vi "acquire multi init subvi ch2.vi"(8 "错误输入（无错误）":errorcluster caption="error in（no error）", 11 "VISA resource name":refnum<visa-resource-name>) -> (0 "错误输出":errorcluster caption="error out", 2 "read buffer":string, 3 "VISA resource name out":refnum<visa-resource-name>)   [LabVIEW 2023, in "owon.lvlib"]
uses:
  owon.lvlib
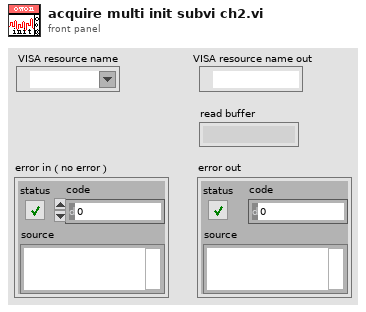
[diagram p1: front panel]
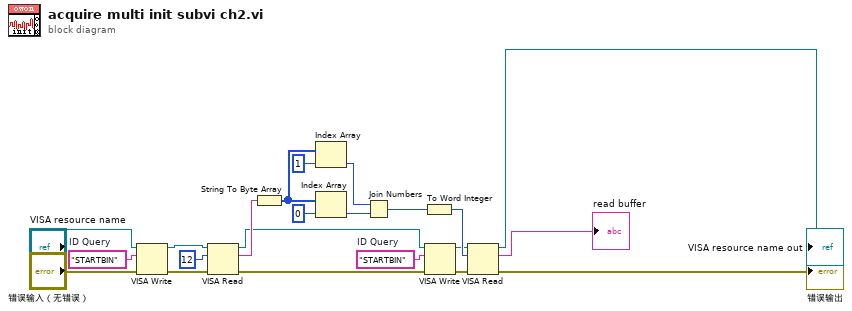
[diagram p0: block diagram]
diagram:
  w14 = "STARTBIN"  # ID Query
  w6 = "STARTBIN"  # ID Query
  n1 = VISA Write(VISA resource name="VISA resource name", write buffer=w14, error in (no error)="错误输入（无错误）") -> (VISA resource name out=w10:refnum<visa-resource-name>, error out=w11:errorcluster)  [unwired: 1 out]
  n2 = VISA Read(VISA resource name=w10, byte count=u32 12, error in (no error)=w11) -> (VISA resource name out=w7:refnum<visa-resource-name>, read buffer=w21:string, error out=w8:errorcluster)  [unwired: 1 out]
  n3 = String To Byte Array(string=w21) -> (unsigned byte array=w16:u8[])
  n4 = Index Array(array=w16, index=1 ("索引")) -> (element=w18:u8)
  n5 = Index Array(array=w16, index=0 ("索引")) -> (element=w19:u8)
  n6 = Join Numbers(hi=w18, lo=w19) -> ((hi.lo)=w20:u16)
  n7 = To Word Integer(number=w20) -> (16bit integer=w22:i16)
  n8 = VISA Write(VISA resource name=w7, write buffer=w6, error in (no error)=w8) -> (VISA resource name out=w3:refnum<visa-resource-name>, error out=w4:errorcluster)  [unwired: 1 out]
  n9 = VISA Read(VISA resource name=w3, byte count=w22, error in (no error)=w4) -> (VISA resource name out=→"VISA resource name out":refnum<visa-resource-name>, read buffer=→"read buffer":string, error out=→"错误输出":errorcluster)  [unwired: 1 out]
